vi "Timer for heating.vi"(8 "shift before":u32) -> (0 "shift after":u32, 2 "Время нагрева":timestamp=timestamp(-10799.222 s since 1904-01-01) format="%<%H:%M:%S>T", 4 "Текущее время":dbl, 5 "Текущее время (array)":dbl[](array[numeric]))   [LabVIEW 2016]
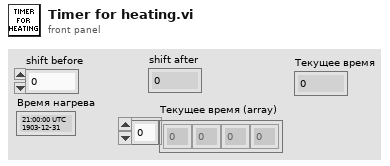
[diagram p1: front panel]
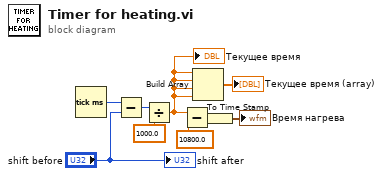
[diagram p0: block diagram]
diagram:
  n1 = Tick Count (ms)() -> (millisecond timer value=w9:u32)
  n2 = Subtract(x=w9, y="shift before") -> (x-y=w7:u32)
  n3 = Divide(x=w7, y=1000.0) -> (x/y=w2:dbl)
  "Текущее время" <- w2
  n4 = Subtract(x=w2, y=10800.0) -> (x-y=w6:dbl)
  n5 = Build Array(w2, w2, w2, w2) -> (→"Текущее время (array)":dbl[])
  n6 = To Time Stamp(1:w6) -> (0:→"Время нагрева":timestamp)
  "shift after" <- "shift before"
